vi "GetTime.vi"(8 "error in (no error)":errorcluster) -> (0 "error out":errorcluster, 1 "TimeInSeconds":i32, 2 "TimeStringForPath":string, 3 "TimeString":string)   [LabVIEW 2014]
panel:
  out "number 4":i32
  out "number 3":i32
  out "number 2":i32
  out "before substring 3":string
  out "before substring 2":string
  out "before substring":string
  out "date string":string
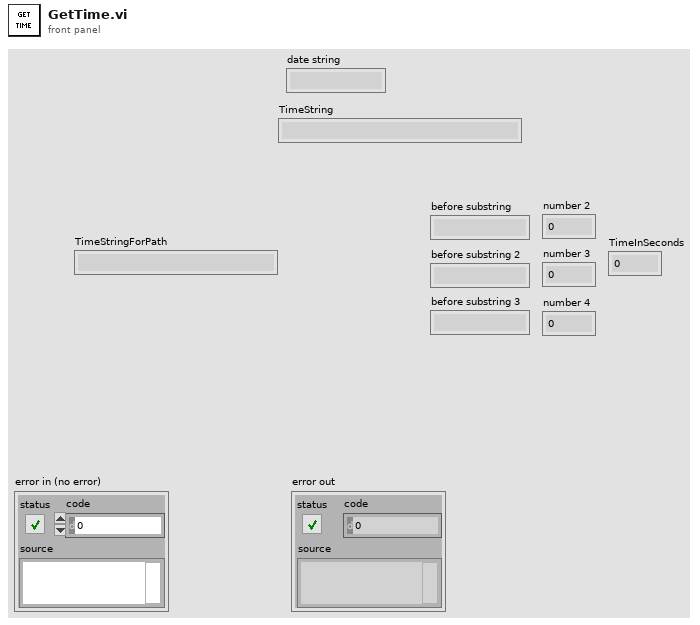
[diagram p1: front panel]
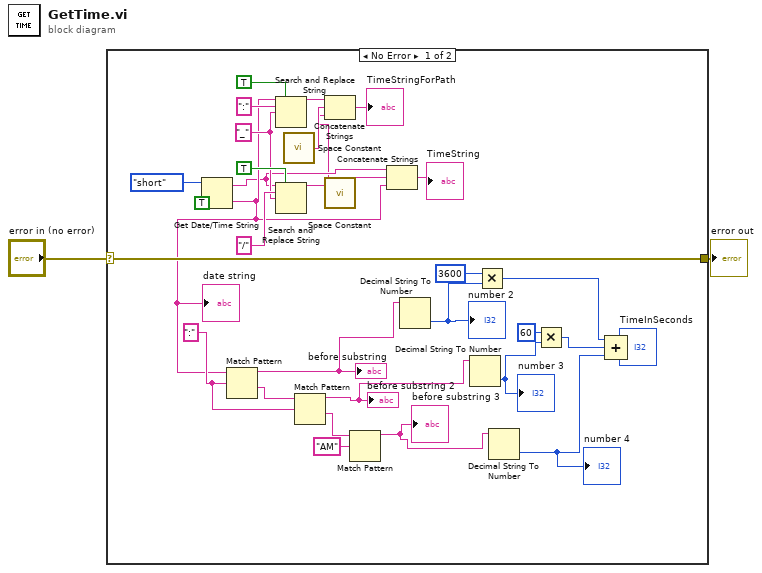
[diagram p0: block diagram]
diagram:
  n1 = case shown="No Error" "error in (no error)" {
    selector: "error in (no error)" -> [w33 w34]
    tunnel: [w33 w34] -> w1
    frame No Error {
      w23 = ":" ("regular expression")
      w26 = "_" ("replace string (\"\")")
      n2 = Get Date/Time String(date format (0)=enum16{"short", "long", "abbreviated"}."short", want seconds? (F)=TRUE) -> (date string=w6:string, time string=w9:string)  [unwired: 1 in]
      "date string" <- w9
      n3 = Match Pattern(string=w9, regular expression=w23) -> (before substring=w20:string, after substring=w24:string)  [unwired: 1 in, 2 out]
      "before substring" <- w20
      n4 = Search and Replace String(replace all?=TRUE ("replace all? (F)"), input string=w9, search string=":", replace string=w26) -> (result string=w3:string)  [unwired: 4 in, 3 out]
      n5 = Search and Replace String(replace all?=TRUE ("replace all? (F)"), input string=w6, search string="/", replace string=w26) -> (result string=w4:string)  [unwired: 4 in, 3 out]
      n6 = call <vilib>:"Space Constant.vi"() -> ("String"=w5:string)
      n7 = Match Pattern(string=w24, regular expression=w23) -> (before substring=w19:string, after substring=w22:string)  [unwired: 1 in, 2 out]
      "before substring 2" <- w19
      n8 = Concatenate Strings(w3, w5, w4) -> (→"TimeStringForPath":string)
      n9 = call <vilib>:"Space Constant.vi"() -> ("String"=w7:string)
      n10 = Match Pattern(string=w22, regular expression="AM") -> (before substring=w18:string)  [unwired: 1 in, 3 out]
      "before substring 3" <- w18
      n11 = Concatenate Strings(w6, w7, w9) -> (→"TimeString":string)
      n12 = Decimal String To Number(string=w20) -> (number=w17:i32)  [unwired: 2 in, 1 out]
      "number 2" <- w17
      n13 = Decimal String To Number(string=w19) -> (number=w15:i32)  [unwired: 2 in, 1 out]
      "number 3" <- w15
      n14 = Multiply(x=3600, y=w17) -> (x*y=w13:i32)
      n15 = Decimal String To Number(string=w18) -> (number=w11:i32)  [unwired: 2 in, 1 out]
      "number 4" <- w11
      n16 = Multiply(x=60, y=w15) -> (x*y=w12:i32)
      n17 = Compound Arithmetic op=ADD(w13, w12, w11) -> (→"TimeInSeconds":i32)
    }
    frame Error {
    }
  }
  "error out" <- w1
